vi "3458read.vi"(11 "Instrument Cluster":T1) -> (0 "Measurement value out":dbl)   [LabVIEW 2013]
uses:
  <vilib>/Utility/error.llb/DialogType.ctl
  <instrlib>/Agilent 3458/Public/Data/Read Measurement(Single Point).vi
  <instrlib>/Agilent 3458/Agilent 3458.lvlib
panel:
  out "Manual Range (1.00) 2":dbl=1.0 format="%_3g"
  out "Auto Range (1:ON)":u16(ring)=1 items=["OFF", "ON", "ONCE"]
  out "Frequency Source (3: AC Voltage)":u16(ring)=3 items=["AC + DC Current", "AC + DC Voltage", "AC Current", "AC Voltage"]
  out "Trigger Type (0:Auto)":u16(ring) items=["Auto", "External", "Level", "Line", "Synchronous"]
  out "Manual Resolution (2: 6.5 digits)":enum16{"4.5", "5.5", "6.5", "7.5", "8.5"}(ring)=enum."8.5"
  out "Function (0: DC Voltage) 2":u16(ring) items=["DC Voltage", "AC Voltage", "AC + DC Voltage", "DC Current", "AC Current", "AC + DC Current", "2-Wire Resistance", "4-Wire Resistance", "Frequency", "Period", "Direct Sampling DC", "Direct Sampling AC"]
  out "after substring":string
  out "find instrument":string[](array[string])=["GPIB0::4::INSTR"]
  out "before substring":string
  in  "VISA resource name":refnum<visa-resource-name>
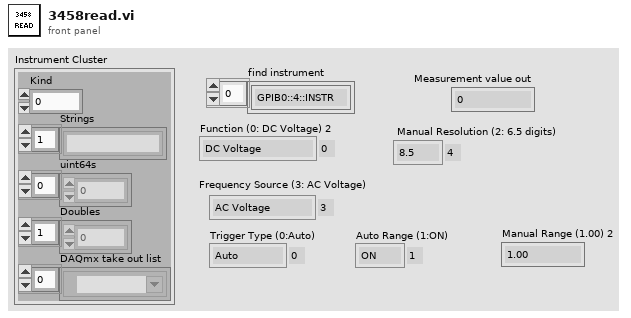
[diagram p1: front panel]
types:
  T1 = cluster{"Kind":u16, "Strings":string[], "uint64s":u64[], "Doubles":dbl[], "DAQmx take out list":refnum<k21>[]}
  T2 = typedef "DialogType.ctl" = u16
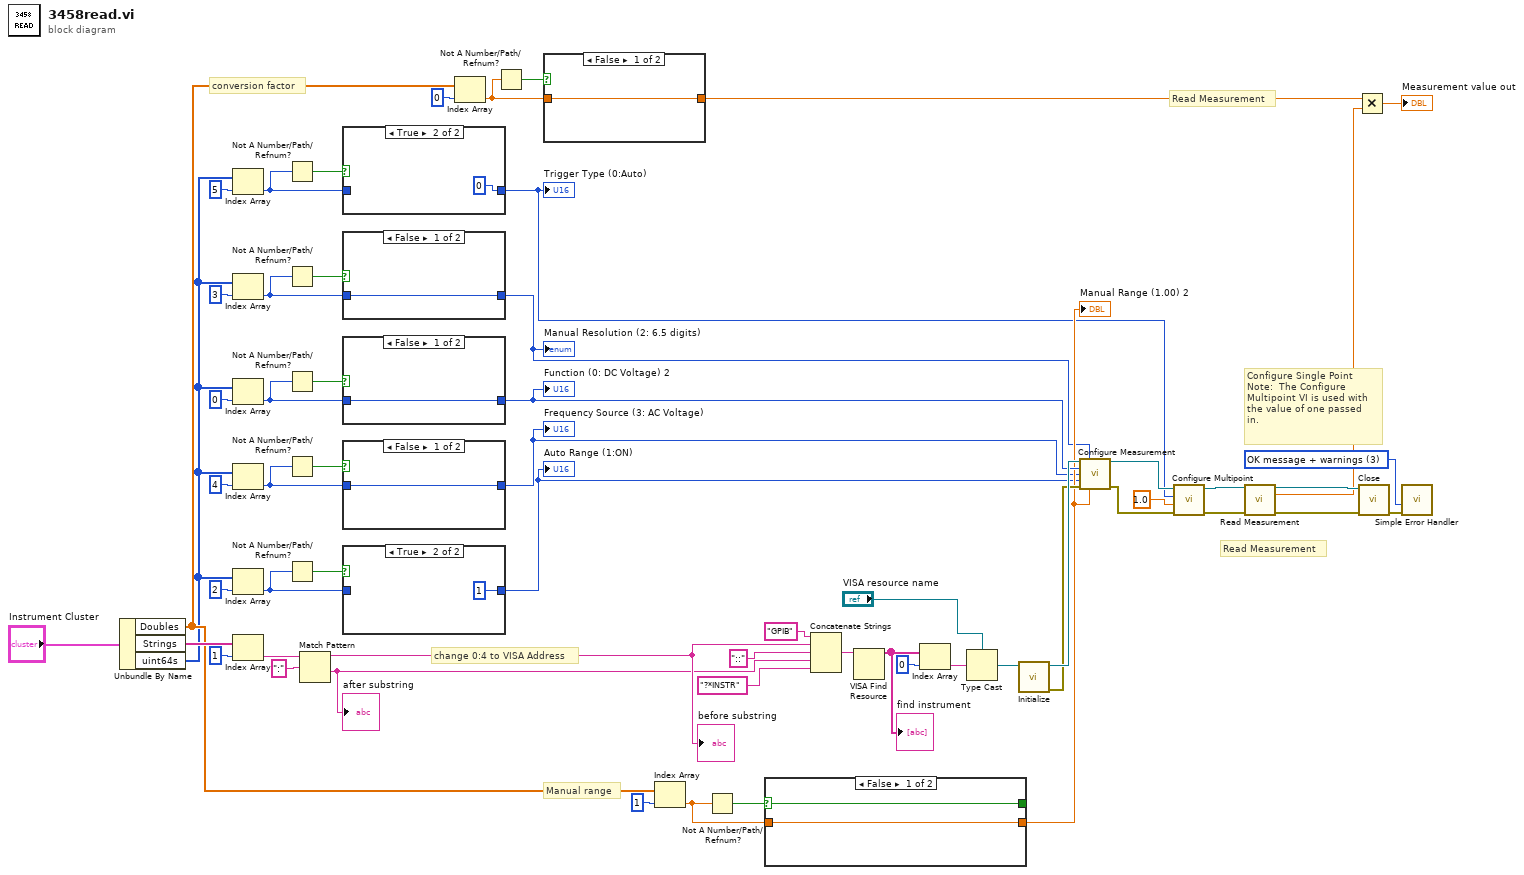
[diagram p0: block diagram]
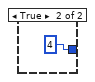
[diagram p3: hidden frame]
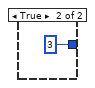
[diagram p5: hidden frame]
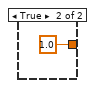
[diagram p6: hidden frame]
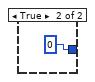
[diagram p7: hidden frame]
diagram:
  w1 = T2 3 items=["no dialog", "OK message", "continue or stop message", "OK message + warnings", "continue/stop + warnings"] ("type of dialog (OK msg:1)")
  # "Configure Single Point\nNote:  The Configure \nMultipoint VI is used with\nthe value of one passed\nin."
  # "Read Measurement"
  # "change 0:4 to VISA Address"
  # "conversion factor"
  # "Manual range"
  # "Read Measurement"
  n1 = Unbundle By Name("Instrument Cluster") -> ("Doubles"=w52:dbl[], "Strings"=w58:string[], "uint64s"=w3:u64[])
  n2 = Index Array(array=w3, index=5) -> (element=w4:u64)
  n3 = Index Array(array=w3, index=3) -> (element=w8:u64)
  n4 = Index Array(array=w3, index=0) -> (element=w48:u64)
  n5 = Index Array(array=w3, index=4) -> (element=w15:u64)
  n6 = Index Array(array=w3, index=2) -> (element=w13:u64)
  n7 = Index Array(array=w58, index=1) -> (element=w43:string)
  n8 = Not A Number/Path/Refnum?(number/path/refnum=w4) -> (NaN/Path/Refnum?=w5:bool)
  n9 = Not A Number/Path/Refnum?(number/path/refnum=w8) -> (NaN/Path/Refnum?=w9:bool)
  n10 = Not A Number/Path/Refnum?(number/path/refnum=w48) -> (NaN/Path/Refnum?=w49:bool)
  n11 = Not A Number/Path/Refnum?(number/path/refnum=w15) -> (NaN/Path/Refnum?=w16:bool)
  n12 = Not A Number/Path/Refnum?(number/path/refnum=w13) -> (NaN/Path/Refnum?=w14:bool)
  n13 = Match Pattern(string=w43, regular expression=":") -> (before substring=w39:string, after substring=w38:string)  [unwired: 1 in, 2 out]
  "before substring" <- w39
  "after substring" <- w38
  n14 = case shown="True" w5 {
    tunnel: [w60 0] -> w2
    tunnel: w4 -> [w60 _]
    frame False {
    }
    frame True {
    }
  }
  "Trigger Type (0:Auto)" <- w2
  n15 = case shown="False" w9 {
    tunnel: [w62 4] -> w7
    tunnel: w8 -> [w62 _]
    frame False {
    }
    frame True {
    }
  }
  "Manual Resolution (2: 6.5 digits)" <- w7
  n16 = case shown="False" w49 {
    tunnel: [w64 0] -> w20
    tunnel: w48 -> [w64 _]
    frame False {
    }
    frame True {
    }
  }
  "Function (0: DC Voltage) 2" <- w20
  n17 = case shown="False" w16 {
    tunnel: [w66 3] -> w11
    tunnel: w15 -> [w66 _]
    frame False {
    }
    frame True {
    }
  }
  "Frequency Source (3: AC Voltage)" <- w11
  n18 = case shown="True" w14 {
    tunnel: [w68 1] -> w12
    tunnel: w13 -> [w68 _]
    frame False {
    }
    frame True {
    }
  }
  "Auto Range (1:ON)" <- w12
  n19 = Index Array(array=w52, index=0) -> (element=w46:dbl)
  n20 = Not A Number/Path/Refnum?(number/path/refnum=w46) -> (NaN/Path/Refnum?=w47:bool)
  n21 = case shown="False" w47 {
    tunnel: [w70 1.0] -> w45
    tunnel: w46 -> [w70 _]
    frame False {
    }
    frame True {
    }
  }
  n22 = Index Array(array=w52, index=1) -> (element=w55:dbl)
  n23 = Not A Number/Path/Refnum?(number/path/refnum=w55) -> (NaN/Path/Refnum?=w56:bool)
  n24 = case shown="False" w56 {
    selector: w56 -> [w73 w74]
    tunnel: [w73 w74] -> _
    tunnel: w55 -> [w72 _]
    tunnel: [w72 _] -> w19
    frame False {
    }
    frame True {
      # "if nan auto range True"
    }
  }
  "Manual Range (1.00) 2" <- w19
  n25 = Concatenate Strings("GPIB", w39, "::", w38, "?*INSTR") -> (w36:string)
  n26 = VISA Find Resource(11:w36) -> (3:w35:string[])  [unwired: 2 in, 2 out]
  "find instrument" <- w35
  n27 = Index Array(array=w35, index=0) -> (element=w33:string)
  n28 = Type Cast(type="VISA resource name", x=w33) -> (*(type *) &x=w22:refnum<visa-resource-name>)
  n29 = call <instrlib>:"Initialize.vi"("VISA resource name"=w22) -> ("error out"=w25:errorcluster, "VISA resource name out"=w26:refnum<visa-resource-name>)  [unwired: 9 in]
  n30 = call <instrlib>:"Configure Measurement.vi"("VISA resource name"=w26, "Manual Resolution (2: 6.5 digits)"=w7, "Function (0: DC Voltage)"=w20, "Frequency Source (3: AC Voltage)"=w11, "Auto Range (1:ON)"=w12, "error in (no error)"=w25, "Manual Range (1.00)"=w19) -> ("VISA resource name out"=w28:refnum<visa-resource-name>, "error out"=w27:errorcluster)  [unwired: 7 in]
  n31 = call <instrlib>:"Configure Multipoint.vi"("error in (no error)"=w27, "Sample Count (1)"=1.0, "Trigger Type (0:Auto)"=w2, "VISA resource name"=w28) -> ("error out"=w23:errorcluster, "VISA resource name out"=w24:refnum<visa-resource-name>)  [unwired: 6 in]
  n32 = call-poly <instrlib>:"Read Measurement.vi"("VISA resource name"=w24, "error in (no error)"=w23) -> ("VISA resource name out"=w31:refnum<visa-resource-name>, "Measurement"=w21:dbl, "error out"=w30:errorcluster)  [unwired: 11 in]
  n33 = Multiply(x=w45, y=w21) -> (x*y=→"Measurement value out":dbl)
  n34 = call <instrlib>:"Close.vi"("error in (no error)"=w30, "VISA resource name"=w31) -> ("error out"=w29:errorcluster)  [unwired: 9 in]
  n35 = call <vilib>:"Simple Error Handler.vi"("type of dialog (OK msg:1)"=w1, "error in (no error)"=w29) -> ()  [unwired: 3 in, 5 out]
